vi "Reset Iterations.vi"(8 "error in (no error)":errorcluster, 11 "Measurement in":refnum<class "Measurement.lvclass">) -> (0 "error out":errorcluster, 3 "Measurement out":refnum<class "Measurement.lvclass">)   [LabVIEW 2015, in "Measurement Actor.lvlib" / "Measurement.lvclass"]
uses:
  Measurement.lvclass
  Measurement.lvclass/Measurement.ctl
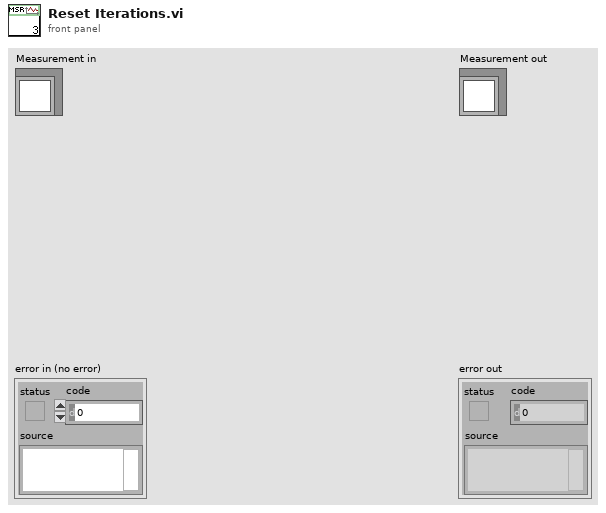
[diagram p1: front panel]
types:
  T1 = typedef "Measurement Actor.lvlib/Measurement.lvclass/Iteration count.ctl" = cluster{"Desired Iterations":i32, "Current":i32}
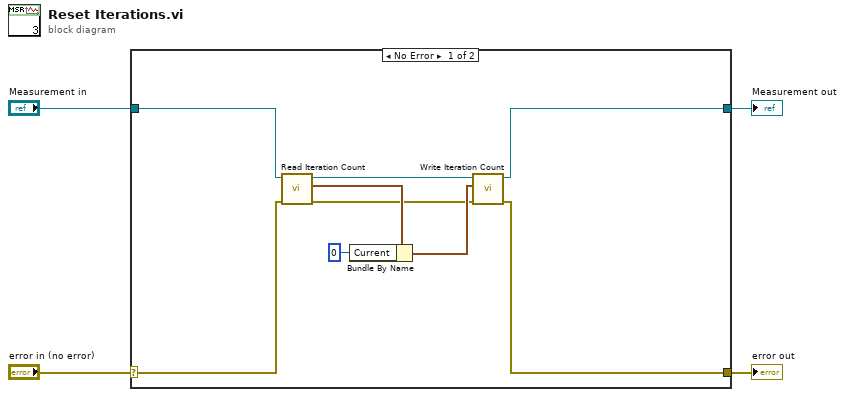
[diagram p0: block diagram]
diagram:
  n1 = case shown="No Error" "error in (no error)" {
    selector: "error in (no error)" -> [w6 w15]
    tunnel: [w5 w15] -> w3
    tunnel: [w8 w14] -> w1
    tunnel: "Measurement in" -> [w9 w14]
    frame No Error {
      n2 = call "Read Iteration Count.vi"("error in (no error)"=w6, "Measurement in"=w9) -> ("error out"=w7:errorcluster, "Iteration Count"=w13:T1, "Measurement out"=w10:refnum<class "Measurement.lvclass">)  [unwired: 7 in]
      n3 = Bundle By Name(cluster=w13, "Current"=0) -> (w11:T1)
      n4 = call "Write Iteration Count.vi"("error in (no error)"=w7, "Iteration Count"=w11, "Measurement in"=w10) -> ("error out"=w5:errorcluster, "Measurement out"=w8:refnum<class "Measurement.lvclass">)  [unwired: 7 in]
    }
    frame Error {
    }
  }
  "error out" <- w3
  "Measurement out" <- w1
